vi "Calculate Vector Distance.vi"(9 "V2":cluster{"x":dbl, "y":dbl}, 10 "V1":cluster{"x":dbl, "y":dbl}) -> (2 "Distance out":dbl)   [LabVIEW 2021, in "Utils.lvlib"]
doc: "MIT Licence\nCopyright (c) 2024 David Grollier"
uses:
  Utils.lvlib
  <vilib>/Analysis/_algsub.llb/Vector Norm Type.ctl
  <vilib>/Analysis/_algsub.llb/Real Vector Norm.vi
  <vilib>/Analysis/NI_AALPro.lvlib
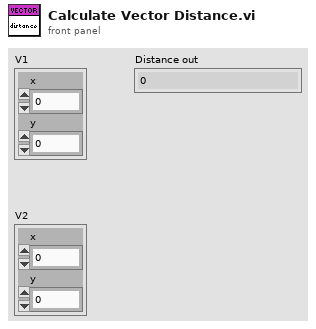
[diagram p1: front panel]
types:
  T1 = typedef "NI_AALPro.lvlib/Vector Norm Type.ctl" = u16
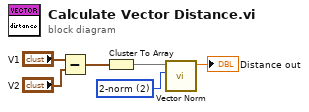
[diagram p0: block diagram]
diagram:
  w5 = T1 2 items=["1-norm"=1, "2-norm"=2, "Inf-norm"=3, "-Inf-norm"=4, "User Defined"=5] ("norm type")
  n1 = Subtract(x="V1", y="V2") -> (x-y=w2:cluster{"x":dbl, "y":dbl})
  n2 = Cluster To Array(cluster=w2) -> (array=w6:dbl[])
  n3 = call-poly <vilib>:"Vector Norm.vi"("norm type"=w5, "Input Vector"=w6) -> ("norm"=→"Distance out":dbl)  [unwired: 8 in, 1 out]
